vi "Returning Values By Reference Pointer To Complex Struct Corrected.vi"(8 "error in (no error)":errorcluster) -> (0 "error out":errorcluster, 3 "triangle out":T2)   [LabVIEW 2009, in "LabVIEWWrapper_PassingDataSampleDLL.lvlib"]
doc: "void ReturningValuesByReference_PointerToComplexStruct (struct complexStructPolygon* triangle);"
uses:
  LabVIEWWrapper_PassingDataSampleDLL.lvlib
  CustomControlsForStructs/ComplexStruct Polygon Pointer.ctl
  CustomControlsForStructs/ComplexStruct Polygon.ctl
  <vilib>/Utility/importsl/GetValueByPointer/GetValueByPointer.xnode
  <vilib>/Utility/importsl/GetValueByPointer/datatype.ctl
  PassingDataSampleDLL.dll
  Program Files (x86)/National Instruments/LabVIEW 2009/resource/lvimptsl.dll
panel:
  out "Output Triangle":T1
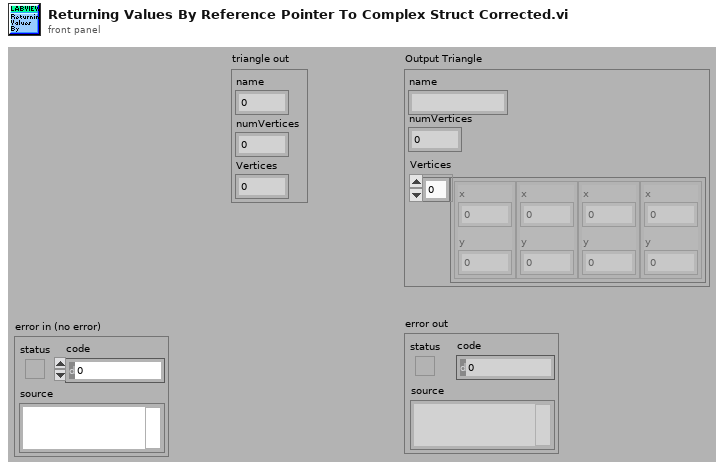
[diagram p1: front panel]
types:
  T1 = typedef "LabVIEWWrapper_PassingDataSampleDLL.lvlib/ComplexStruct Polygon.ctl" = cluster{"name":string, "numVertices":i32, "Vertices":cluster{"x":i32, "y":i32}[]}
  T2 = typedef "LabVIEWWrapper_PassingDataSampleDLL.lvlib/ComplexStruct Polygon Pointer.ctl" = cluster{"name":u32, "numVertices":i32, "Vertices":i32}
  T3 = cluster{"name":u32, "numVertices":i32, "Vertices":i32}
  T4 = cluster{"Output":string, "numVertices":i32, cluster{"Output":i32, "Output":i32}[]}
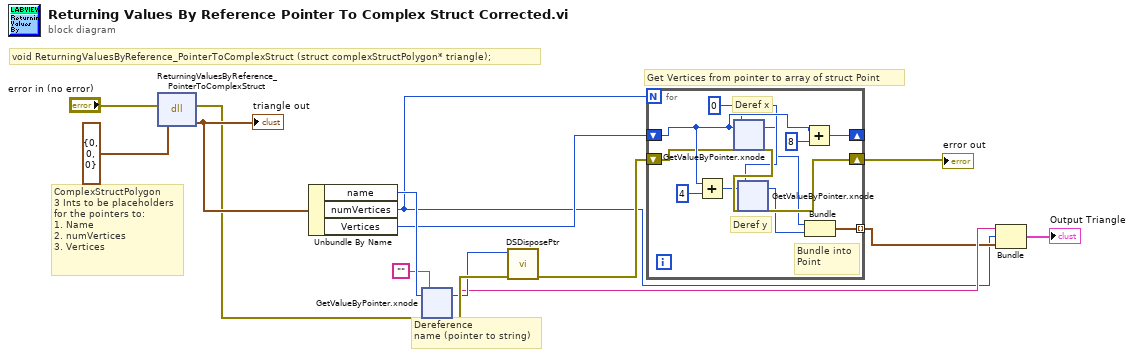
[diagram p0: block diagram]
diagram:
  # "Get Vertices from pointer to array of struct Point"
  # "Dereference\nname (pointer to string)"
  # "ComplexStructPolygon\n3 Ints to be placeholders\nfor the pointers to:\n1. Name\n2. numVertices\n3. Vertices"
  # "void ReturningValuesByReference_PointerToComplexStruct (struct complexStructPolygon* triangle);"
  n1 = dll-call lib="C:/My Dropbox/Systems Engineering Application/SDK/C Integration/LabVIEWWrapper/PassingDataSampleDLL.*" fn="ReturningValuesByReference_PointerToComplexStruct"(error in="error in (no error)", T3 {"name"=0, "numVertices"=0, "Vertices"=0} ("triangle")) -> (error out=w6:errorcluster, w7:T3)  [unwired: 3 in, 1 out]
  "triangle out" <- w7
  n2 = Unbundle By Name(w7) -> ("name"=w13:u32, "numVertices"=w1:i32, "Vertices"=w10:i32)
  n3 = xnode "GetValueByPointer.xnode"("Pointer"=w13, "InputType"="", "ErrorIn"=w6) -> ("Output"=w3:string, "ErrorOut"=w14:errorcluster)  [unwired: 1 in]
  n4 = call <vilib>:"DSDisposePtr.vi"("error in (no error)"=w14, "Pointer"=w13) -> ("error out"=w9:errorcluster)  [unwired: 9 in]
  n5 = for {
    N: w1 -> [_]
    shift-right: [w21] -> _
    shift-left: w10 -> [w22]
    shift-right: [w19] -> w5
    shift-left: w9 -> [w20]
    tunnel: [w15] -> w2 mode=indexing
    w18 = 0
    # "Deref y"
    # "Deref x"
    # "Bundle into\nPoint"
    n6 = Add(x=w22, y=4) -> (x+y=w25:i32)
    n7 = xnode "GetValueByPointer.xnode"("Pointer"=w22, "InputType"=w18, "ErrorIn"=w20) -> ("Output"=w17:i32, "ErrorOut"=w26:errorcluster)  [unwired: 1 in]
    n8 = xnode "GetValueByPointer.xnode"("Pointer"=w25, "InputType"=w18, "ErrorIn"=w26) -> ("Output"=w16:i32, "ErrorOut"=w19:errorcluster)  [unwired: 1 in]
    n9 = Add(x=w22, y=8) -> (x+y=w21:i32)
    n10 = Bundle("Output"=w17, "Output"=w16) -> (w15:cluster{"Output":i32, "Output":i32})  [unwired: 1 in]
  }
  "error out" <- w5
  n11 = Bundle("Output"=w3, "numVertices"=w1, w2) -> (→"Output Triangle":T4)  [unwired: 1 in]
